vi "COPIE.vi"() -> ()   [LabVIEW 2013]
panel:
  out "data 2":dynamicdata(graph) caption="données"
  out "Fréquence":dbl
  in  "Frequence de Echantillonage (khz)":dbl
  in  "Voie":enum16{"AI0", "AI2", "AI4", "AI6"}(ring)
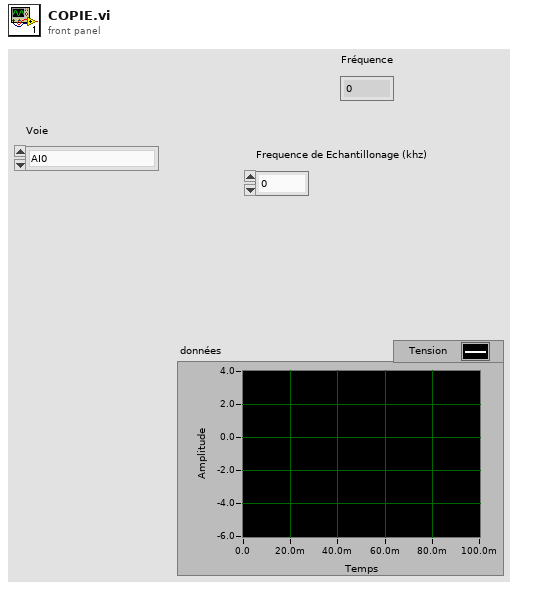
[diagram p1: front panel]
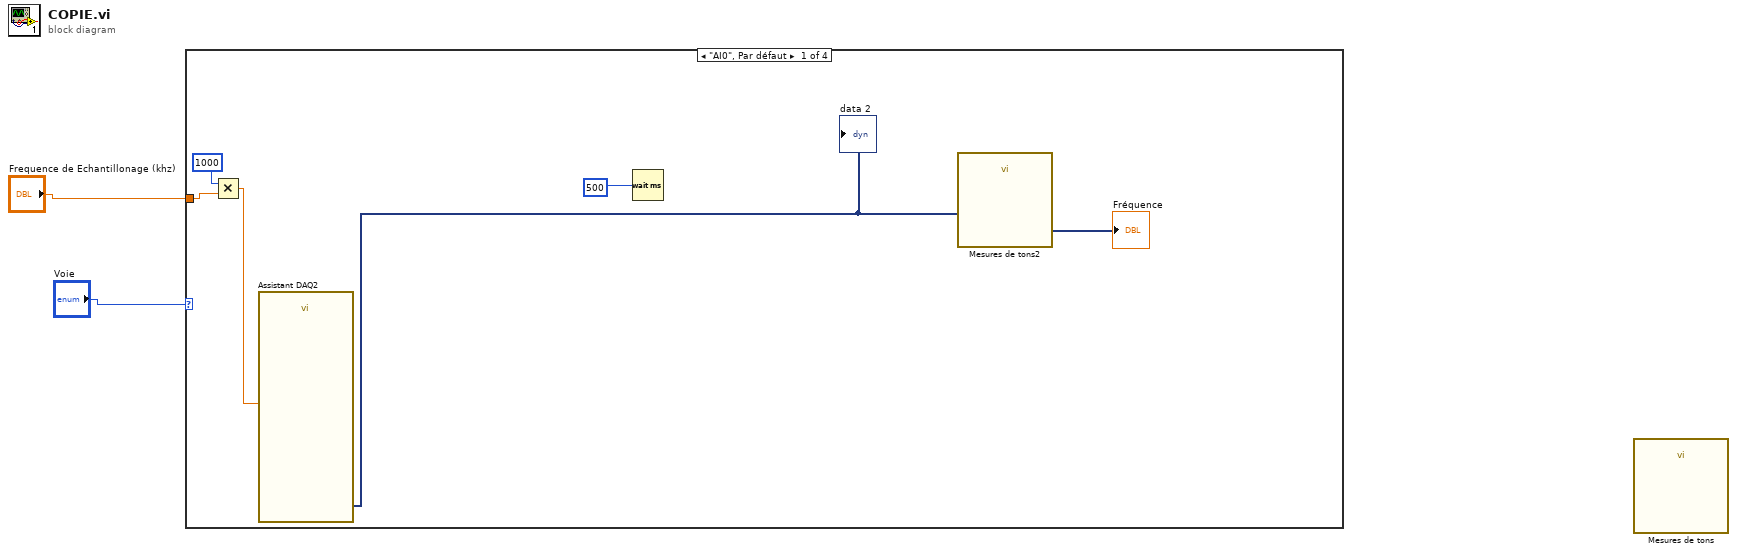
[diagram p0: block diagram]
diagram:
  n1 = case shown="\"AI0\", Par défaut" "Voie" {
    tunnel: "Frequence de Echantillonage (khz)" -> [w8 _ _ _]
    frame "AI0", Default {
      n2 = Multiply(x=1000, y=w8) -> (x*y=w6:dbl)
      n3 = call "Assistant DAQ2"("vitesse"=w6) -> ("data"=w3:dynamicdata)  [unwired: 16 in, 2 out]
      "data 2" <- w3
      n4 = Wait (ms)(milliseconds to wait=500) -> ()  [unwired: 1 out]
      n5 = call "Mesures de tons2"("Signals"=w3) -> ("Frequency"=→"Fréquence":dynamicdata)  [unwired: 9 in, 1 out]
    }
    frame "AI2" {
    }
    frame "AI4" {
    }
    frame "AI6" {
    }
  }
  n6 = call "Mesures de tons"() -> ()  [unwired: 10 in, 2 out]
